vi "Send Error Task_Manager.vi"(8 "error in (no error)":errorcluster, 11 "Error Task Manager in":refnum<class "Error Task Manager.lvclass">) -> (0 "error out":errorcluster, 3 "Error Task Manager out":refnum<class "Error Task Manager.lvclass">)   [LabVIEW 2013, in "Error Task Manager.lvlib" / "Error Task Manager.lvclass"]
doc: "This vi Send Task Manager Error"
uses:
  Error Task Manager.lvclass
  Error Task Manager.lvclass/Error Task Manager.ctl
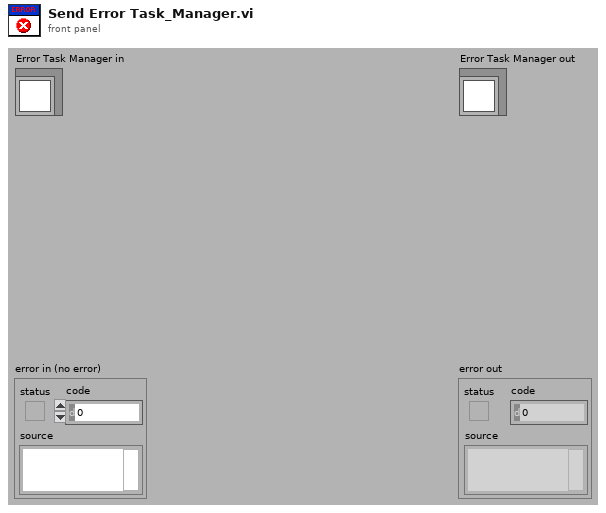
[diagram p1: front panel]
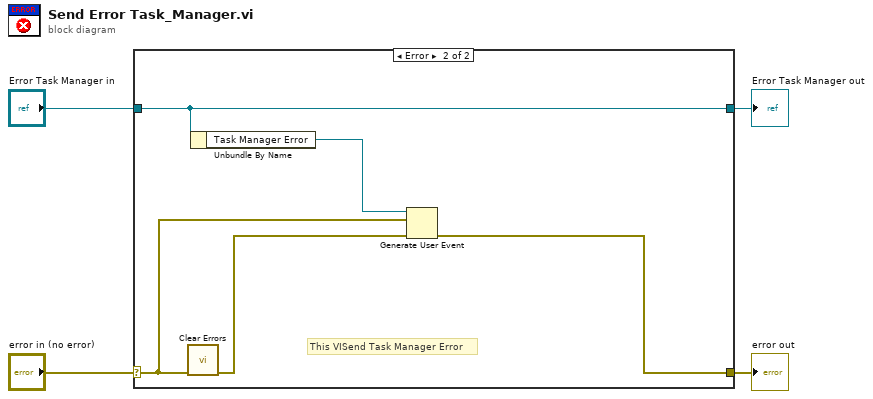
[diagram p0: block diagram]
diagram:
  n1 = case shown="Error" "error in (no error)" {
    selector: "error in (no error)" -> [w6 w9]
    tunnel: [w6 w7] -> w3
    tunnel: [w5 w11] -> w1
    tunnel: "Error Task Manager in" -> [w5 w11]
    frame No Error {
    }
    frame Error {
      # "This VISend Task Manager Error"
      n2 = call <vilib>:"Clear Errors.vi"("error in (no error)"=w9) -> ("error out"=w8:errorcluster)  [unwired: 6 in]
      n3 = Unbundle By Name(w11) -> ("Task Manager Error"=w10:refnum<user-event>)
      n4 = Generate User Event(user event=w10, event data cluster=w9, error in=w8) -> (error out=w7:errorcluster)  [unwired: 1 in, 1 out]
    }
  }
  "error out" <- w3
  "Error Task Manager out" <- w1
